vi "16_12_Fxp_addation.vi"(1 "y":fxp<+/-,12,16>, 2 "x":fxp<+/-,12,16>) -> (0 "x+y":fxp<+/-,13,17> format="%.41g")   [LabVIEW 2020]
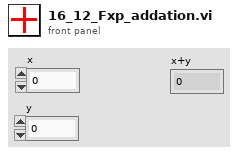
[diagram p1: front panel]
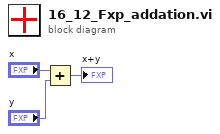
[diagram p0: block diagram]
diagram:
  n1 = Add(x="x", y="y") -> (x+y=→"x+y":fxp<+/-,13,17>)
